vi "Aquire Image.vi"(8 "error in (no error)":errorcluster, 9 "Cluster":T1={"Gamma::Value"=1.6, "Gain::Value"=50, "Sharpness::Value"=0, "Contrast::Value"=0.5, "Exposure::Value"=0.0078125} {"Exposure::Value" min=0.000244140625 max=0.5; "Contrast::Value" min=0.0 max=1.0; "Sharpness::Value" min=0 max=2 step=1; "Gain::Value" min=0 max=100 step=1; "Gamma::Value" min=0.01 max=10.0}, 10 "Stop":bool, 11 "Camera in":refnum<class "Camera.lvclass">) -> (0 "error out":errorcluster, 2 "Image Out":T2(plugin-control), 3 "Camera out":refnum<class "Camera.lvclass">)   [LabVIEW 2018, in "Camera.lvclass"]
uses:
  Camera.lvclass
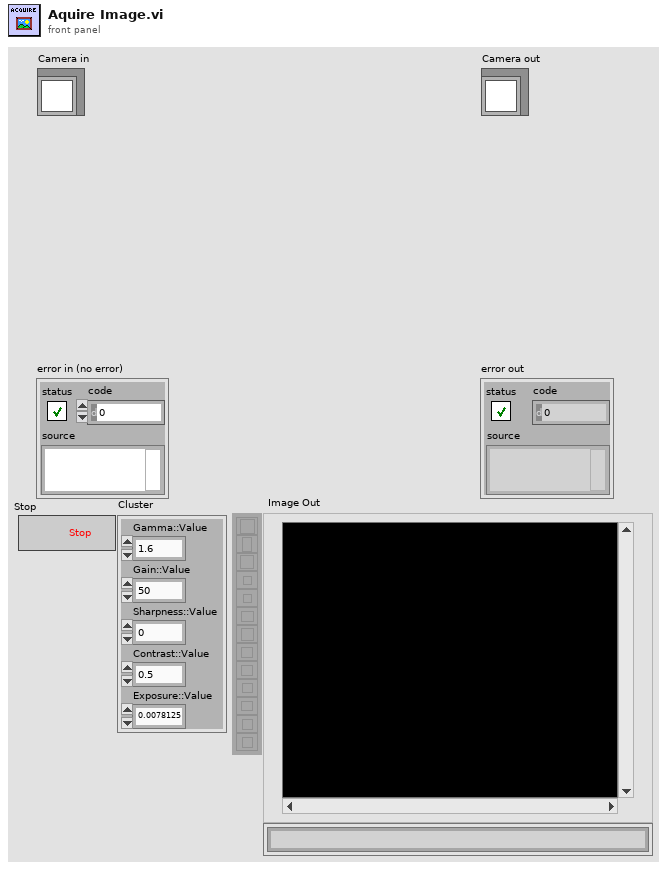
[diagram p1: front panel]
types:
  T1 = cluster{"Gamma::Value":dbl, "Gain::Value":i64, "Sharpness::Value":i64, "Contrast::Value":dbl, "Exposure::Value":dbl}
  T2 = typedef "IMAQ Image.ctl" = refnum<image>
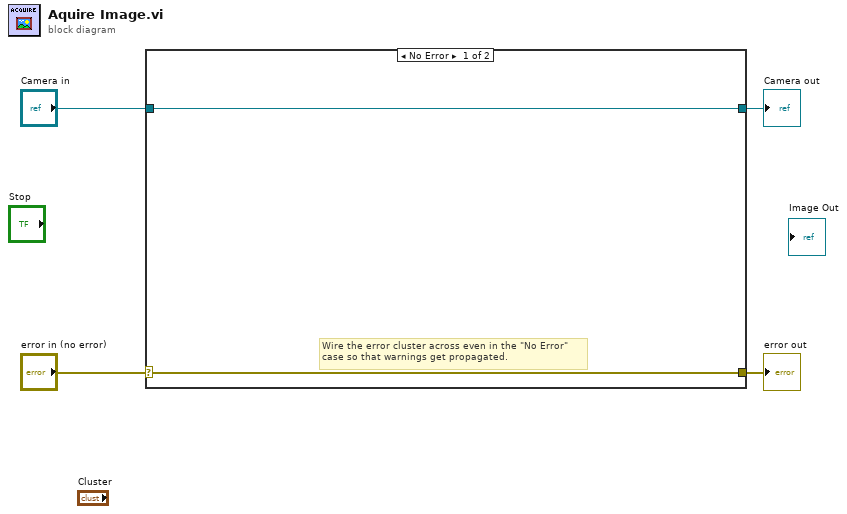
[diagram p0: block diagram]
diagram:
  n1 = case shown="No Error" "error in (no error)" {
    selector: "error in (no error)" -> [w5 w8]
    tunnel: [w5 w8] -> w3
    tunnel: [w6 w7] -> w1
    tunnel: "Camera in" -> [w6 w7]
    frame No Error {
      # "Wire the error cluster across even in the \"No Error\"\ncase so that warnings get propagated."
    }
    frame Error {
    }
  }
  "error out" <- w3
  "Camera out" <- w1
